vi "Get Boolean.vi"(1 "Name":string) -> (0 "Value":bool)   [LabVIEW 2016]
doc: "Used to retrieve boolean values for use in \"until\" subcommands."
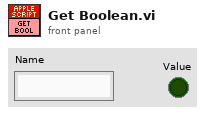
[diagram p1: front panel]
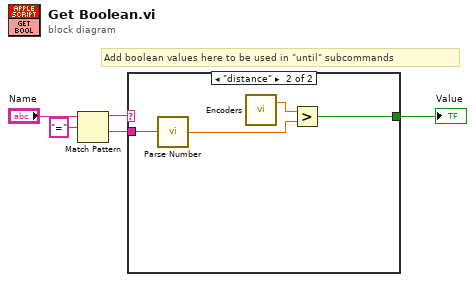
[diagram p0: block diagram]
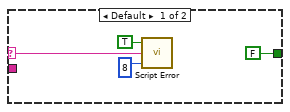
[diagram p2: hidden frame]
diagram:
  # "Add boolean values here to be used in \"until\" subcommands"
  n1 = Match Pattern(string="Name", regular expression="=") -> (before substring=w3:string, after substring=w1:string)  [unwired: 1 in, 2 out]
  n2 = case shown="\"distance\"" w3 {
    selector: w3 -> [w6 _]
    tunnel: [FALSE w10] -> w5
    tunnel: w1 -> [_ w12]
    frame Default {
      n3 = call "Script Error.vi"("Error?"=TRUE, "Error Details"=w6, "Error Code"=8) -> ()  [unwired: 2 in, 1 out]
    }
    frame "distance" {
      n4 = call "Parse Number.vi"("String"=w12) -> ("Number"=w11:dbl)
      n5 = call "Encoders.vi"() -> ("Avg Absolute Distance"=w13:dbl)  [unwired: 2 in, 1 out]
      n6 = Greater?(x=w13, y=w11) -> (0:w10:bool)
    }
  }
  "Value" <- w5
